vi "physiology_panel.vi"() -> ()   [LabVIEW 2015]
panel:
  in  "Use Opto Stim":bool
  out "Opto Stim":waveform(dbl)[](graph) caption="Opto Stim Display"
  out "700B Primary":waveform(dbl)[](graph) caption="700B Primary Display"
  out "vi_prop_err":errorcluster
  in  "stop_button":bool
  # "Read in from master panel"
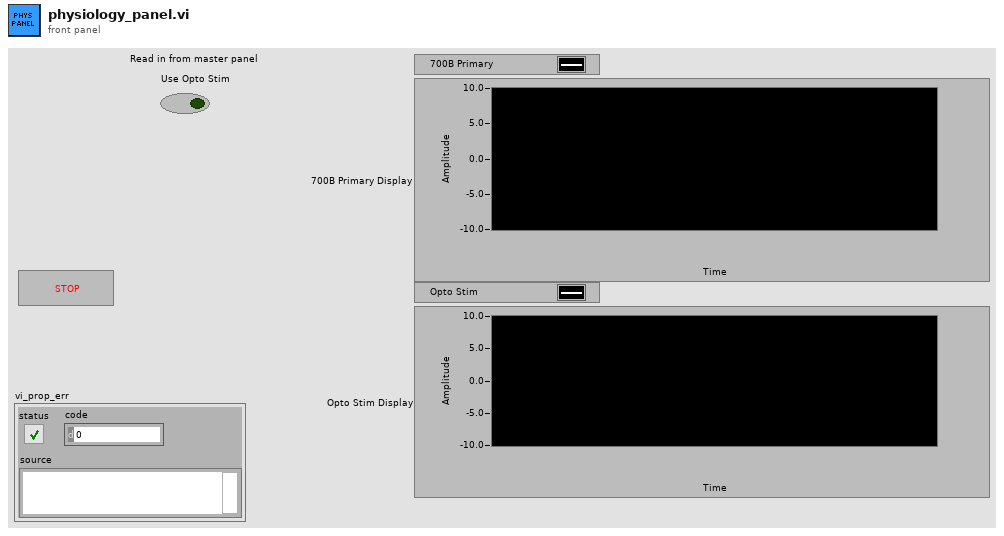
[diagram p1: front panel]
types:
  T1 = enum32{"Invalid", "Standard", "Closed", "Hidden", "Minimized", "Maximized"}
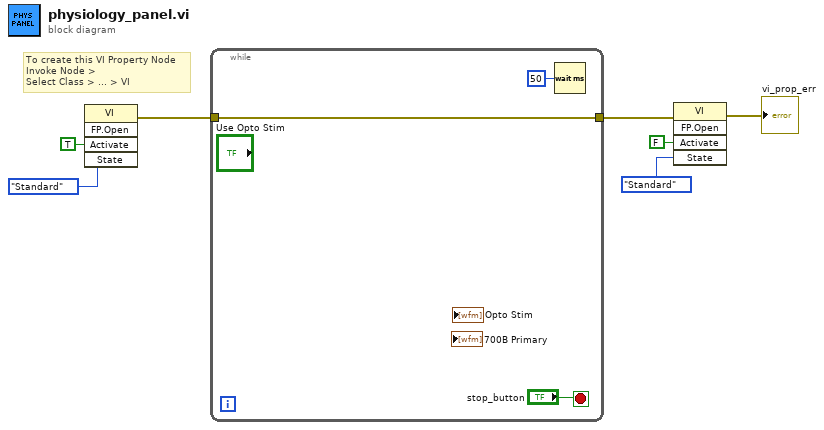
[diagram p0: block diagram]
diagram:
  # "To create this VI Property Node \nInvoke Node >\nSelect Class > ... > VI"
  n1 = invoke class="VI" method="FP.Open"("Activate"=TRUE ("Activate?"), "State"=T1."Standard") -> (error out=w5:errorcluster)  [unwired: 3 in, 4 out]
  n2 = while {
    tunnel: w5 -> [w9]
    tunnel: [w9] -> w4
    stop <- "stop_button" stop-if-true
    n3 = Wait (ms)(milliseconds to wait=u32 50) -> ()  [unwired: 1 out]
  }
  n4 = invoke class="VI" method="FP.Open"(error in=w4, "Activate"=FALSE ("Activate?"), "State"=T1."Standard") -> (error out=→"vi_prop_err":errorcluster)  [unwired: 2 in, 4 out]
